vi "DFConfig Write Crawldir Config.vi"(0 "Datafinder Search Area":T1={"path"=path "", "remotepath"=path "", "alias"="", "volatile"=TRUE, "type"="favorite", "lastcrawl"=timestamp(0 s since 1904-01-01), "numberofcrawls"=0, "crawlnow"=FALSE}, 3 "Config In":string, 4 "Tag (\"\")":string) -> (5 "Config Out":string)   [LabVIEW 2011]
uses:
  DFConfig SEARCH AREA.ctl
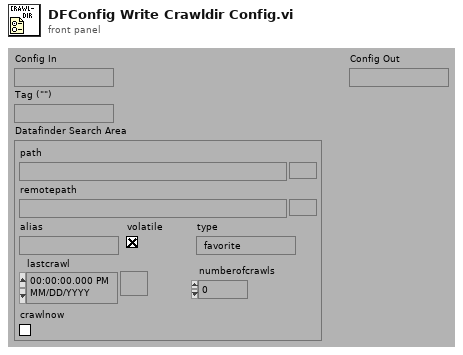
[diagram p1: front panel]
types:
  T1 = typedef "DFConfig SEARCH AREA.ctl" = cluster{"path":path, "remotepath":path, "alias":string, "volatile":bool, "type":string, "lastcrawl":timestamp, "numberofcrawls":i32, "crawlnow":bool}
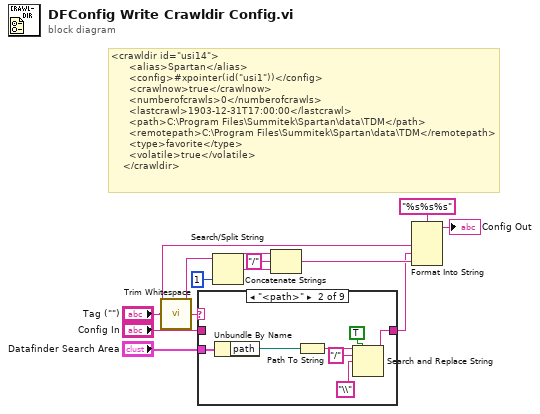
[diagram p0: block diagram]
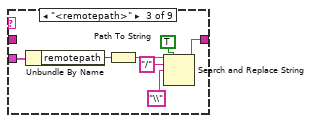
[diagram p3: hidden frame]
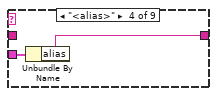
[diagram p4: hidden frame]
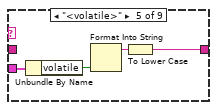
[diagram p5: hidden frame]
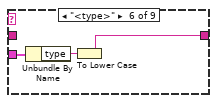
[diagram p6: hidden frame]
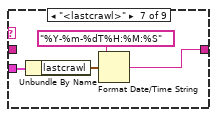
[diagram p7: hidden frame]
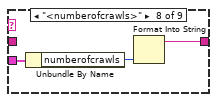
[diagram p8: hidden frame]
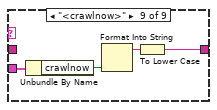
[diagram p9: hidden frame]
diagram:
  # "<crawldir id=\"usi14\">\n      <alias>Spartan</alias>\n      <config>#xpointer(id(\"usi1\"))</config>\n      <crawlnow>true</crawlnow>\n      <numberofcrawls>0</numberofcrawls>\n      <lastcrawl>1903-12-31T17:00:00</lastcrawl>\n      <path>C:\\Program Files\\Summitek\\Spartan\\data\\TDM</path>\n      <remotepath>C:\\Program Files\\Summitek\\Spartan\\data\\TDM</remotepath>\n      <type>favorite</type>\n      <volatile>true</volatile>\n    </crawldir>"
  n1 = call <vilib>:"Trim Whitespace.vi"("string"="Tag (\"\")") -> ("trimmed string"=w1:string)  [unwired: 1 in]
  n2 = case shown="\"<path>\"" w1 {
    tunnel: "Datafinder Search Area" -> [_ w20 w27 w29 w33 w36 w40 w43 w47]
    tunnel: [w13 w14 w21 w28 w30 w35 w39 w41 w44] -> w4
    tunnel: "Config In" -> [w13 _ _ _ _ _ _ _ _]
    frame "<NOP>", Default {
    }
    frame "<path>" {
      n3 = Unbundle By Name(w20) -> ("path"=w15:path)
      n4 = Path To String(path=w15) -> (string=w16:string)
      n5 = Search and Replace String(replace all?=TRUE ("replace all? (F)"), input string=w16, search string="/", replace string="\\" ("replace string (\"\")")) -> (result string=w14:string)  [unwired: 1 in, 6 out]
    }
    frame "<remotepath>" {
      n6 = Unbundle By Name(w27) -> ("remotepath"=w26:path)
      n7 = Path To String(path=w26) -> (string=w22:string)
      n8 = Search and Replace String(replace all?=TRUE ("replace all? (F)"), input string=w22, search string="/", replace string="\\" ("replace string (\"\")")) -> (result string=w21:string)  [unwired: 1 in, 6 out]
    }
    frame "<alias>" {
      n9 = Unbundle By Name(w29) -> ("alias"=w28:string)
    }
    frame "<volatile>" {
      n10 = Unbundle By Name(w33) -> ("volatile"=w32:bool)
      n11 = Format Into String(w32) -> (resulting string=w31:string)  [unwired: 3 in, 1 out]
      n12 = To Lower Case(string=w31) -> (all lower case string=w30:string)
    }
    frame "<type>" {
      n13 = Unbundle By Name(w36) -> ("type"=w34:string)
      n14 = To Lower Case(string=w34) -> (all lower case string=w35:string)
    }
    frame "<lastcrawl>" {
      n15 = Unbundle By Name(w40) -> ("lastcrawl"=w38:timestamp)
      n16 = Format Date/Time String(time format string (%c)="%Y-%m-%dT%H:%M:%S", seconds (now)=w38) -> (date/time string=w39:string)  [unwired: 1 out]
    }
    frame "<numberofcrawls>" {
      n17 = Unbundle By Name(w43) -> ("numberofcrawls"=w42:i32)
      n18 = Format Into String(w42) -> (resulting string=w41:string)  [unwired: 3 in, 1 out]
    }
    frame "<crawlnow>" {
      n19 = Unbundle By Name(w47) -> ("crawlnow"=w46:bool)
      n20 = Format Into String(w46) -> (resulting string=w45:string)  [unwired: 3 in, 1 out]
      n21 = To Lower Case(string=w45) -> (all lower case string=w44:string)
    }
  }
  n22 = Search/Split String(string=w1, offset (0)=1) -> (substring before match=w8:string, match + rest of string=w7:string)  [unwired: 2 out]
  n23 = Concatenate Strings(w8, "/" ("string"), w7) -> (w6:string)
  n24 = Format Into String(format string="%s%s%s", "Tag (\"\")", w4, w6) -> (resulting string=→"Config Out":string)  [unwired: 2 in, 1 out]
